vi "GetSampleTime.vi"(10 "CellPosition":T1, 11 "MulticolumnListbox输入":refnum<vi>) -> (2 "Area_name":string, 3 "SampleTime":string)   [LabVIEW 2014, in "cyy.lvlib" / "LeakageFenXi.lvlib"]
uses:
  LeakageFenxi/LeakageFenXi.lvlib
  <vilib>/Utility/miscctls.llb/LVRowAndColumnTypeDef.ctl
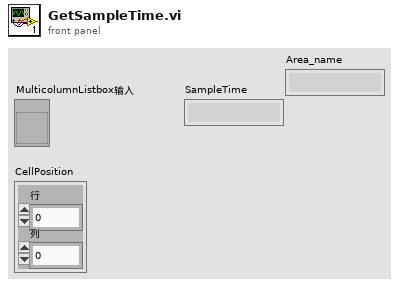
[diagram p1: front panel]
types:
  T1 = typedef "LVRowAndColumnTypeDef.ctl" = cluster{"Row":i32, "Column":i32}
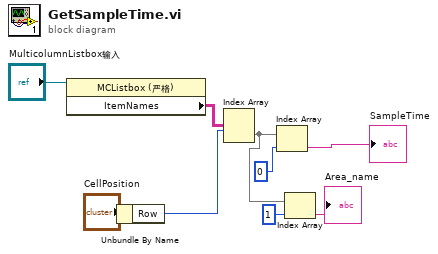
[diagram p0: block diagram]
diagram:
  n1 = property on="属性节点" class="MCListbox (严格)"(reference="MulticolumnListbox输入") -> ("ItemNames"=w6:string[][])  [unwired: 1 in, 2 out]
  n2 = Unbundle By Name("CellPosition") -> ("Row"=w9:i32)
  n3 = Index Array(array=w6, index (row)=w9) -> (element=w3:string[])  [unwired: 1 in]
  n4 = Index Array(array=w3, index=0 ("索引")) -> (element=→"SampleTime":string)
  n5 = Index Array(array=w3, index=1 ("索引")) -> (element=→"Area_name":string)
